vi "Calculate Scenic Scores.vi"(1 "Tree Grid":i32[][](array[numeric])) -> (0 "Scenic Scores":map{cdb, i32}(c390))   [LabVIEW 2020, in "AoC 2022.lvlib"]
uses:
  AoC 2022.lvlib
panel:
  out "Debug: Score Distribution":map{cdb, string}(c390)
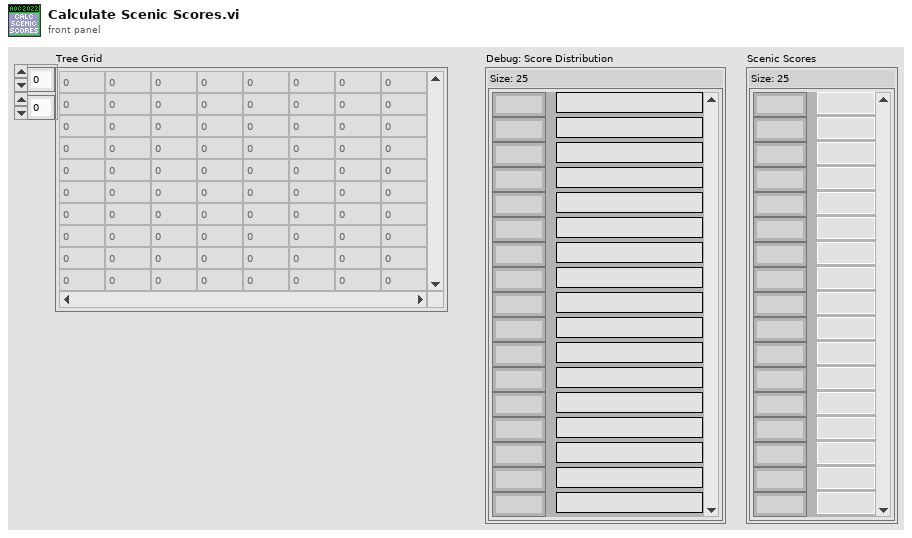
[diagram p1: front panel]
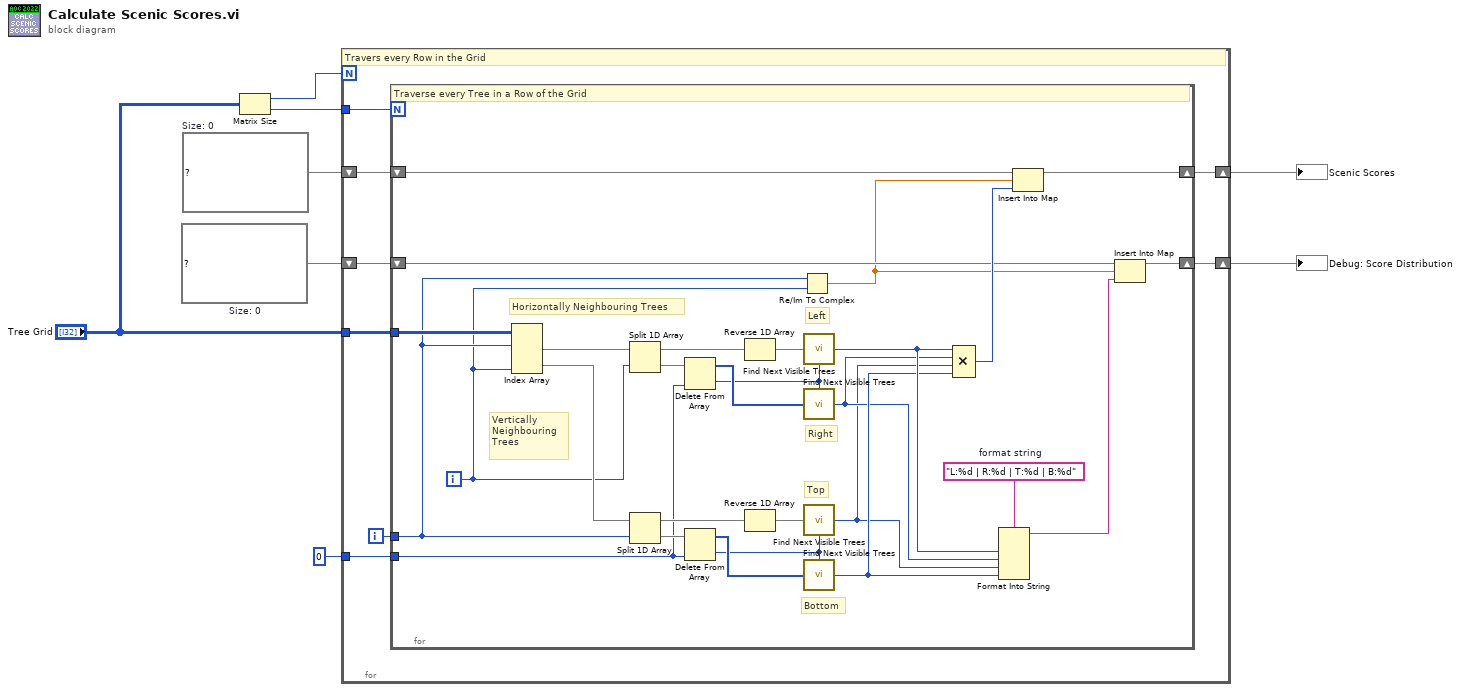
[diagram p0: block diagram]
diagram:
  w6 = map{cdb, string} {}  # Size: 0
  w8 = map{cdb, i32} {}  # Size: 0
  n1 = Matrix Size(0:"Tree Grid") -> (1:w3:i32, 2:w2:i32)
  n2 = for {
    N: w3 -> [_]
    tunnel: "Tree Grid" -> [w16]
    shift-right: [w13] -> w7
    shift-left: w8 -> [w14]
    shift-right: [w11] -> w5
    shift-left: w6 -> [w12]
    tunnel: w2 -> [w10]
    tunnel: 0 -> [w9]
    i -> [w15]
    # "Travers every Row in the Grid"
    n3 = for {
      N: w10 -> [_]
      tunnel: w16 -> [w44]
      tunnel: w15 -> [w31]
      shift-right: [w28] -> w13
      shift-left: w14 -> [w29]
      shift-right: [w24] -> w11
      shift-left: w12 -> [w26]
      tunnel: w9 -> [w17]
      i -> [w30]
      w21 = "L:%d | R:%d | T:%d | B:%d"  # format string
      # "Vertically Neighbouring Trees"
      # "Horizontally Neighbouring Trees"
      # "Bottom"
      # "Top"
      # "Right"
      # "Left"
      # "Traverse every Tree in a Row of the Grid"
      n4 = Index Array(array=w44, index (row) #1=w31, index (col) #2=w30) -> (element #1=w43:i32[], element #2=w33:i32[])  [unwired: 2 in]
      n5 = Split 1D Array(array=w43, index=w30) -> (first subarray=w41:i32[], second subarray=w42:i32[])
      n6 = Split 1D Array(array=w33, index=w31) -> (first subarray=w35:i32[], second subarray=w34:i32[])
      n7 = Delete From Array(array=w42, index=w17) -> (deleted portion=w38:i32, array with subset deleted=w39:i32[])  [unwired: 1 in]
      n8 = Delete From Array(array=w34, index=w17) -> (deleted portion=w32:i32, array with subset deleted=w37:i32[])  [unwired: 1 in]
      n9 = Reverse 1D Array(array=w41) -> (reversed array=w40:i32[])
      n10 = Reverse 1D Array(array=w35) -> (reversed array=w36:i32[])
      n11 = Re/Im To Complex(1:w30, 2:w31) -> (0:w25:cdb)
      n12 = call "Find Next Visible Trees.vi"("Next Trees"=w40, "Current Tree"=w38) -> ("#Next Visible Trees"=w23:i32)
      n13 = call "Find Next Visible Trees.vi"("Next Trees"=w39, "Current Tree"=w38) -> ("#Next Visible Trees"=w19:i32)
      n14 = call "Find Next Visible Trees.vi"("Next Trees"=w36, "Current Tree"=w32) -> ("#Next Visible Trees"=w18:i32)
      n15 = call "Find Next Visible Trees.vi"("Next Trees"=w37, "Current Tree"=w32) -> ("#Next Visible Trees"=w22:i32)
      n16 = Compound Arithmetic op=MULTIPLY(w23, w19, w18, w22) -> (w27:i32)
      n17 = Format Into String(format string=w21, w23, w19, w18, w22) -> (resulting string=w20:string)  [unwired: 2 in, 1 out]
      n18 = Insert Into Map(map in=w29, key=w25, value=w27) -> (map out=w28:map{cdb, i32})  [unwired: 2 out]
      n19 = Insert Into Map(map in=w26, key=w25, value=w20) -> (map out=w24:map{cdb, string})  [unwired: 2 out]
    }
  }
  "Scenic Scores" <- w7
  "Debug: Score Distribution" <- w5
